vi "produceTriggerPulse.vi"(8 "error in (no error)":errorcluster, 10 "Channel":refnum<class "Channel.lvclass">, 11 "device in":refnum<class "device.lvclass">) -> (0 "error out":errorcluster, 3 "device out":refnum<class "device.lvclass">)   [LabVIEW 2009, in "Tools.lvlib" / "DatabaseHelpers.lvlib" / "device.lvclass"]
uses:
  device.lvclass
  Channel/Channel.lvclass
  device.lvclass/device.ctl
  Scripting/ScriptingEvent/ScriptEventList/ScriptEventList.lvclass
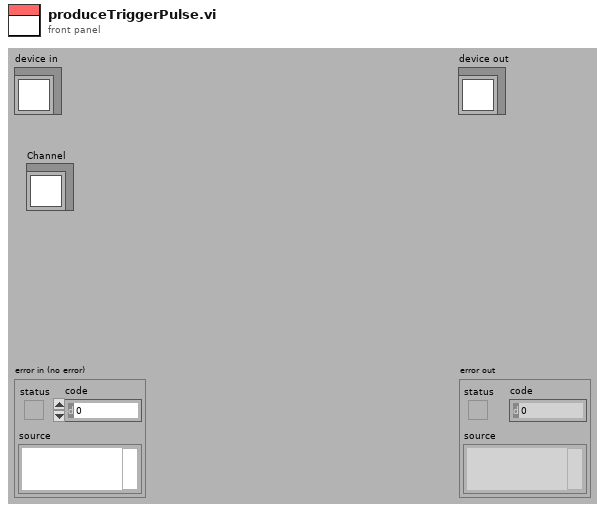
[diagram p1: front panel]
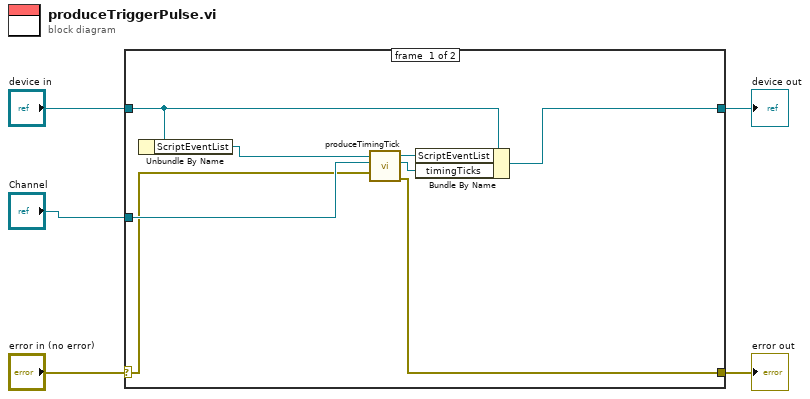
[diagram p0: block diagram]
diagram:
  n1 = case shown="No Error" "error in (no error)" {
    selector: "error in (no error)" -> [w6 w15]
    tunnel: [w10 w15] -> w1
    tunnel: [w12 w14] -> w2
    tunnel: "device in" -> [w13 w14]
    tunnel: "Channel" -> [w9 _]
    frame #0 {
      n2 = Unbundle By Name(w13) -> ("ScriptEventList"=w7:refnum<class "ScriptEventList.lvclass">)
      n3 = call "produceTimingTick.vi"("error in (no error)"=w6, "Channel"=w9, "ScriptEventList in"=w7) -> ("error out"=w10:errorcluster, "timingTick"=w11:refnum<class "ScriptEventList.lvclass">, "ScriptEventList out"=w8:refnum<class "ScriptEventList.lvclass">)  [unwired: 6 in]
      n4 = Bundle By Name(cluster=w13, "ScriptEventList"=w8, "timingTicks"=w11) -> (w12:refnum<class "device.lvclass">)
    }
    frame #1 {
    }
  }
  "error out" <- w1
  "device out" <- w2
